vi "find fit -- set up complex region - V2.vi"(7 "scale factor":dbl=1.0) -> (3 "complex region":T1)   [LabVIEW 2015]
uses:
  complex region.ctl
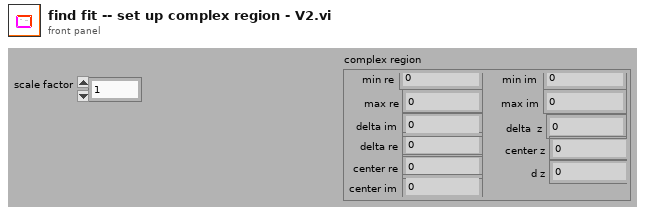
[diagram p1: front panel]
types:
  T1 = typedef "complex region.ctl" = cluster{"max re":dbl, "min re":dbl, "max im":dbl, "min im":dbl, "delta re":dbl, "delta im":dbl, "center re":dbl, "delta  z":cdb, "center im":dbl, "center z":cdb, "d im":dbl, "d re":dbl, "d z":cdb}
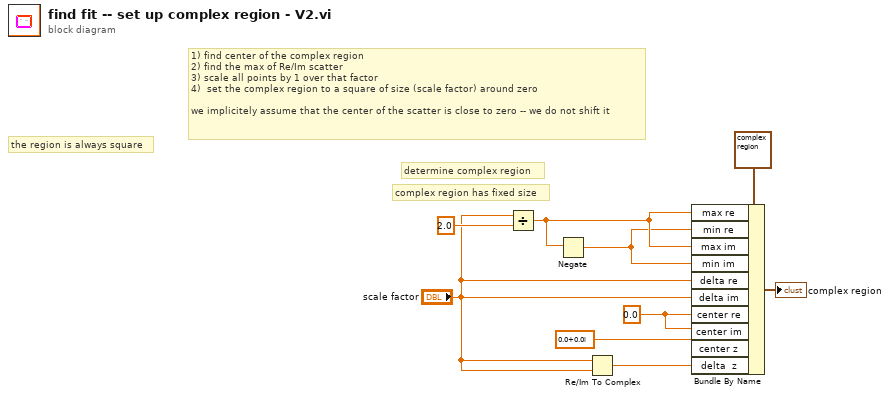
[diagram p0: block diagram]
diagram:
  w2 = 0.0
  # "complex region has fixed size"
  # "1) find center of the complex region\n2) find the max of Re/Im scatter \n3) scale all points by 1 over that factor\n4)  set the complex region to a square of size (scale factor) around zero\n\nwe implicitely assume that the center of the scatter is close to zero -- we do not shift it"
  # "the region is always square"
  # "determine complex region"
  n1 = Divide(x="scale factor", y=2.0) -> (x/y=w5:dbl)
  n2 = Negate(x=w5) -> (-x=w4:dbl)
  n3 = Re/Im To Complex(1:"scale factor", 2:"scale factor") -> (0:w7:cdb)
  n4 = Bundle By Name(cluster=T1 {"max re"=0.0, "min re"=0.0, "max im"=0.0, "min im"=0.0, "delta re"=0.0, "delta im"=0.0, "center re"=0.0, "delta  z"=0.0+0.0i, "center im"=0.0, "center z"=0.0+0.0i, "d im"=0.0, "d re"=0.0, "d z"=0.0+0.0i} ("complex region"), "max re"=w5, "min re"=w4, "max im"=w5, "min im"=w4, "delta re"="scale factor", "delta im"="scale factor", "center re"=w2, "center im"=w2, "center z"=cdb 0.0+0.0i ("x + iy"), "delta  z"=w7) -> (→"complex region":T1)
